vi "test_udp_discovery_client.vi"() -> ()   [LabVIEW 2019]
panel:
  out "rdata":string
  in  "정지":bool
  out "n":i32
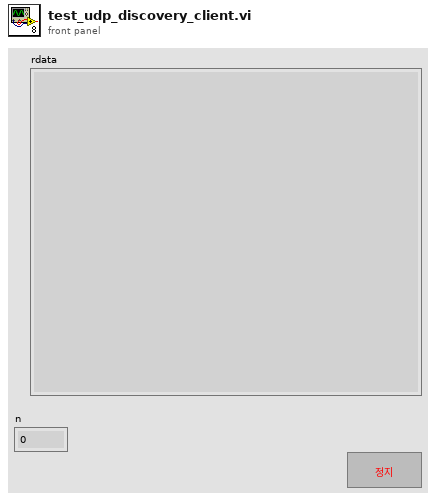
[diagram p1: front panel]
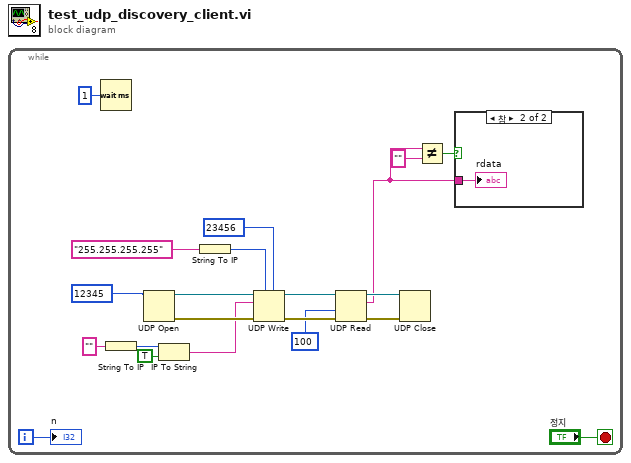
[diagram p0: block diagram]
diagram:
  n1 = while {
    i -> [w5]
    stop <- "정지" stop-if-true
    n2 = Wait (ms)(milliseconds to wait=u32 1 ("대기 시간 (ms)")) -> ()  [unwired: 1 out]
    n3 = String To IP(1:"" ("name")) -> (0:w11:u32)
    n4 = UDP Open(11:u16 12345 ("port")) -> (port=w19:refnum<k16>, 0:w18:errorcluster)  [unwired: 4 in, 1 out]
    n5 = IP To String(1:TRUE ("dot notation? (F)"), 2:w11) -> (0:w9:string)
    n6 = String To IP(1:"255.255.255.255" ("name")) -> (0:w20:u32)
    n7 = UDP Write(address=w20, port or service name=u16 23456 ("port"), connection ID=w19, data in=w9, 8:w18) -> (error out=w15:errorcluster, 3:w16:refnum<k16>)  [unwired: 1 in]
    n8 = UDP Read(connection ID=w16, timeout ms (25000)=100, 8:w15) -> (data out=w2:string, error out=w13:errorcluster, 3:w14:refnum<k16>)  [unwired: 1 in, 2 out]
    n9 = UDP Close(connection ID=w14, 8:w13) -> ()  [unwired: 2 out]
    n10 = Not Equal?(x=w2, y="") -> (x != y?=w3:bool)
    n11 = case shown="참" w3 {
      tunnel: w2 -> [_ w22]
      frame False {
      }
      frame True {
        "rdata" <- w22
      }
    }
    "n" <- w5
  }
